vi "Graph_Data.vi"(8 "error in (no error)":errorcluster, 10 "total_dp_inh2o":dbl[](array[numeric]), 11 "Mass Flow (lbm/min) vs. Pressure Drop (inH2O) - Real Data":dbl[][](array[numeric])) -> (0 "error out":errorcluster, 3 "Model Validation":cluster{dbl[], dbl[]}[](array[cluster]))   [LabVIEW 2025]
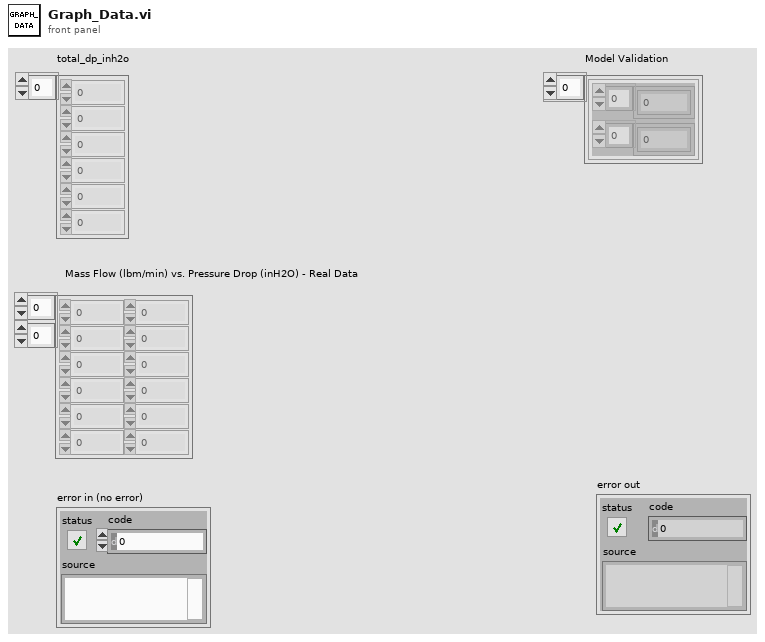
[diagram p1: front panel]
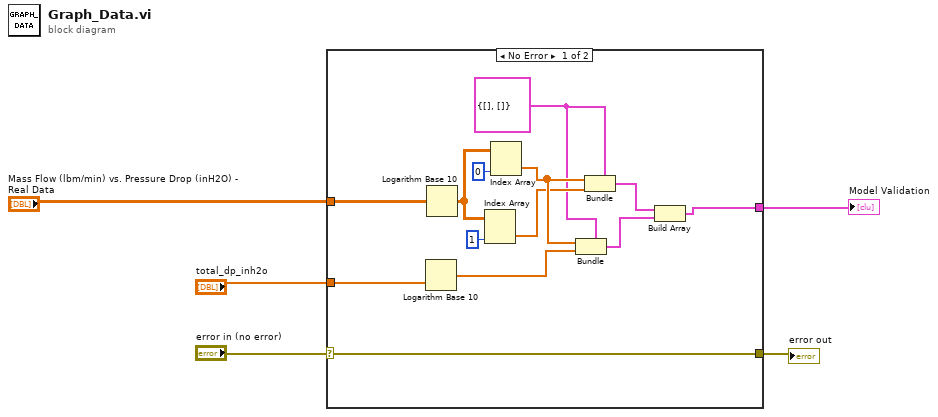
[diagram p0: block diagram]
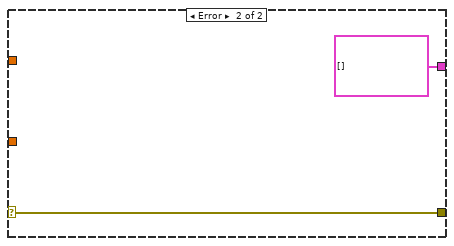
[diagram p2: hidden frame]
diagram:
  n1 = case shown="No Error" "error in (no error)" {
    selector: "error in (no error)" -> [w7 w20]
    tunnel: "Mass Flow (lbm/min) vs. Pressure Drop (inH2O) - Real Data" -> [w18 _]
    tunnel: "total_dp_inh2o" -> [w17 _]
    tunnel: [w7 w20] -> w2
    tunnel: [w6 cluster{dbl[], dbl[]}[] []] -> w1
    frame No Error {
      w8 = cluster{dbl[], dbl[]} {[], []} ("cluster")
      n2 = Logarithm Base 10(1:w17) -> (0:w15:dbl[])
      n3 = Logarithm Base 10(1:w18) -> (0:w9:dbl[][])
      n4 = Index Array(array=w9, index (col)=1 ("disabled index (col)")) -> (element=w14:dbl[])  [unwired: 1 in]
      n5 = Index Array(array=w9, index (col)=0 ("disabled index (col)")) -> (element=w16:dbl[])  [unwired: 1 in]
      n6 = Bundle(cluster=w8, w16, w15) -> (w13:cluster{dbl[], dbl[]})
      n7 = Bundle(cluster=w8, w16, w14) -> (w10:cluster{dbl[], dbl[]})
      n8 = Build Array(w10, w13) -> (w6:cluster{dbl[], dbl[]}[])
    }
    frame Error {
    }
  }
  "error out" <- w2
  "Model Validation" <- w1
